vi "Wireless Logging Example.vi"() -> ()   [LabVIEW 2024]
uses:
  Log Levels.ctl
  Failure Information.ctl
  Log Record.ctl
  Logger/Internal Log Levels.ctl
  ff44e4a9-c346-414c-ae2a-efcf3ff82913.vi
  0679c0b6-e665-4267-8d21-5c2f63ff0cfc.vi
  b68c178a-45ff-4a43-8ee1-f997d7190e6c.vi
  26cdefab-9c11-46d6-bea8-26d872e8373c.vi
  cd3cbcb6-eea4-4d7a-90d3-75033959401d.vi
  3aace37d-2631-4088-b4d1-fd5fc03c86bc.vi
  0679c0b6-e665-4267-8d21-5c2f63ff0cfc.vi/a153a250-4fb8-4a99-bb5b-6ccb57f1f631.vi
  b68c178a-45ff-4a43-8ee1-f997d7190e6c.vi/a02c6254-97f5-44e3-a3a9-7fdb6dfbd055.vi
  26cdefab-9c11-46d6-bea8-26d872e8373c.vi/bae24b8d-f663-491e-8374-2218e527d0d0.vi
  cd3cbcb6-eea4-4d7a-90d3-75033959401d.vi/bf655d3c-1ce4-400f-a78f-0f3f0191886e.vi
  Mark Error.vi
  3aace37d-2631-4088-b4d1-fd5fc03c86bc.vi/ba94d47b-0e30-4c32-b8ff-86d609cd95a5.vi
  0679c0b6-e665-4267-8d21-5c2f63ff0cfc.vi/a153a250-4fb8-4a99-bb5b-6ccb57f1f631.vi/28727e37-b0d9-407c-a479-ab0b7779cd69.vi
  b68c178a-45ff-4a43-8ee1-f997d7190e6c.vi/a02c6254-97f5-44e3-a3a9-7fdb6dfbd055.vi/7453dcce-b283-4a0d-ab92-51c518b086c4.vi
  26cdefab-9c11-46d6-bea8-26d872e8373c.vi/bae24b8d-f663-491e-8374-2218e527d0d0.vi/083db1d9-8cf1-45e4-a540-e8e178cc7cc8.vi
  Handlers/String Handler/String Handler.lvclass
  Formatters/JSON/JSON.lvclass
  <vilib>/Utility/error.llb/Error Cluster From Error Code.vi
  Registry/Enable All.vi
  Registry/Disable All.vi
  Registry/Log.vi
  <vilib>/ErrorRing/Error Ring.xnode
  C:/Users/Colin/Documents/software_projects/glog/Logging/Handlers/Formatting Handler/Formatting Handler.lvclass
  C:/Users/Colin/Documents/software_projects/glog/Logging/Handlers/String Handler/String Handler.lvclass
  Logging.lvlib
  C:/Users/Colin/Documents/software_projects/glog/Logging/Formatters/Formatter/Formatter.lvclass
  C:/Users/Colin/Documents/software_projects/glog/Logging/Formatters/JSON/JSON.lvclass
panel:
  in  "Failure Type":bool
  out "failures info":T1[](array[typedef]) {"Log Record"."timestamp" format="%<%x %.3X>T"}
  in  "error/warning iteration":i32=20
  in  "log messages 2":string
  in  "loop iteration delay [ms]":u32=10
  in  "minimum log level":T4=enum."Info"
  out "error out":errorcluster
  in  "log messages":string
  in  "total iterations":i32=30
  in  "restart logging at":i32=20
  in  "stop logging at":i32=10
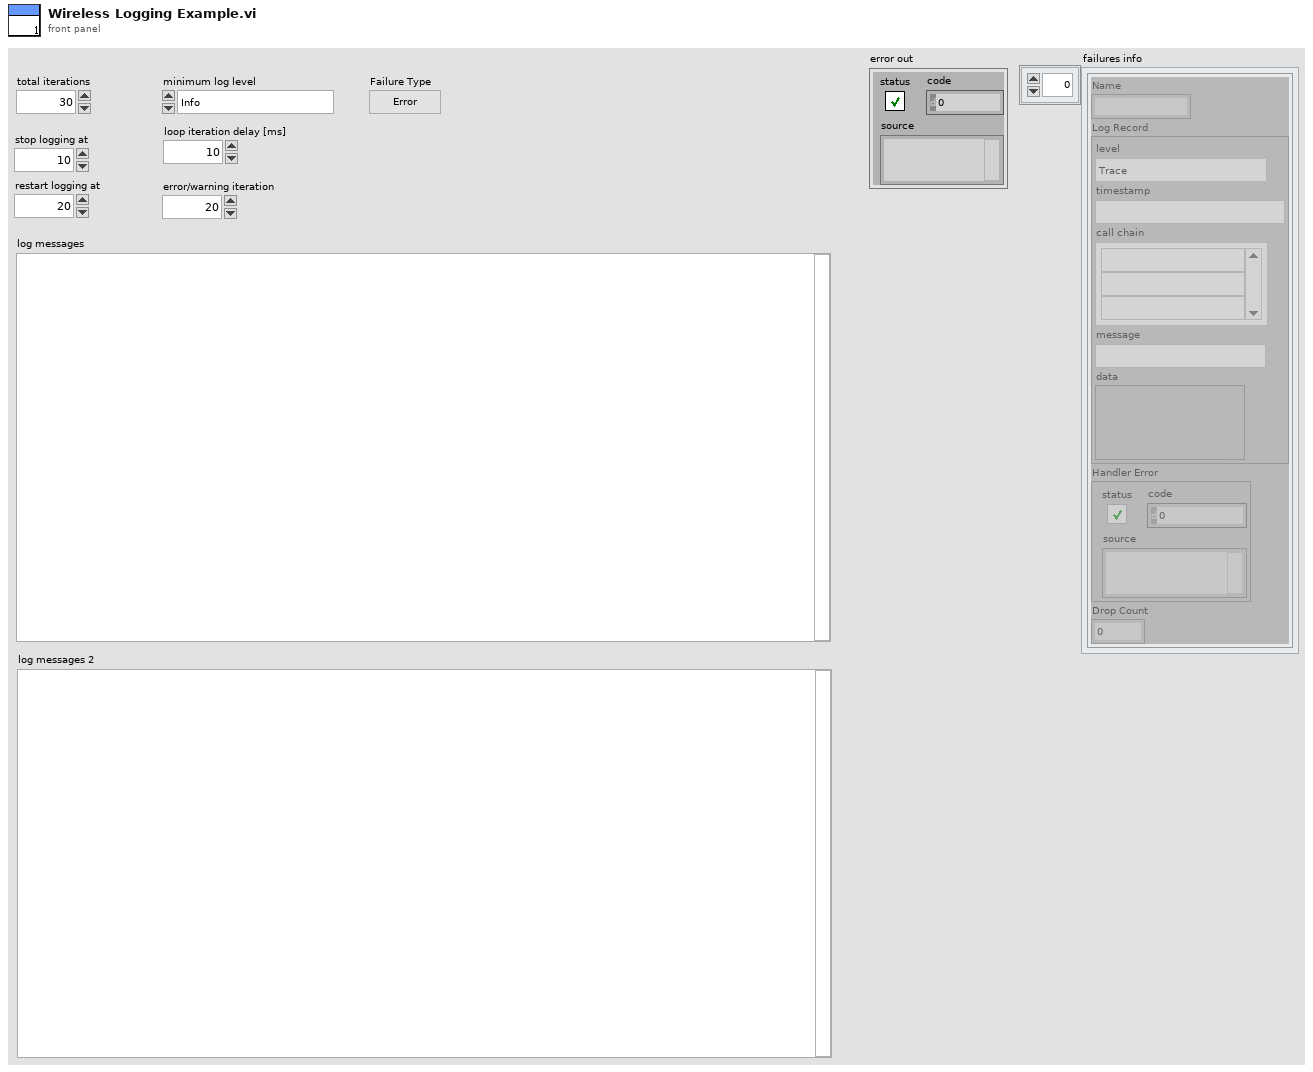
[diagram p1: front panel]
types:
  T1 = typedef "Logging.lvlib/Failure Information.ctl" = cluster{"Name":string, "Log Record":T2, "Handler Error":errorcluster, "Drop Count":u32}
  T2 = typedef "Logging.lvlib/Log Record.ctl" = cluster{"level":T3, "timestamp":timestamp, "call chain":string[], "message":string, "data":variant}
  T3 = typedef "Logging.lvlib/Internal Log Levels.ctl" = enum16{"Trace", "Debug", "Info", "Warning", "Error", "Critical", "Internal"}
  T4 = typedef "Logging.lvlib/Log Levels.ctl" = enum16{"Trace", "Debug", "Info", "Warning", "Error", "Critical"}
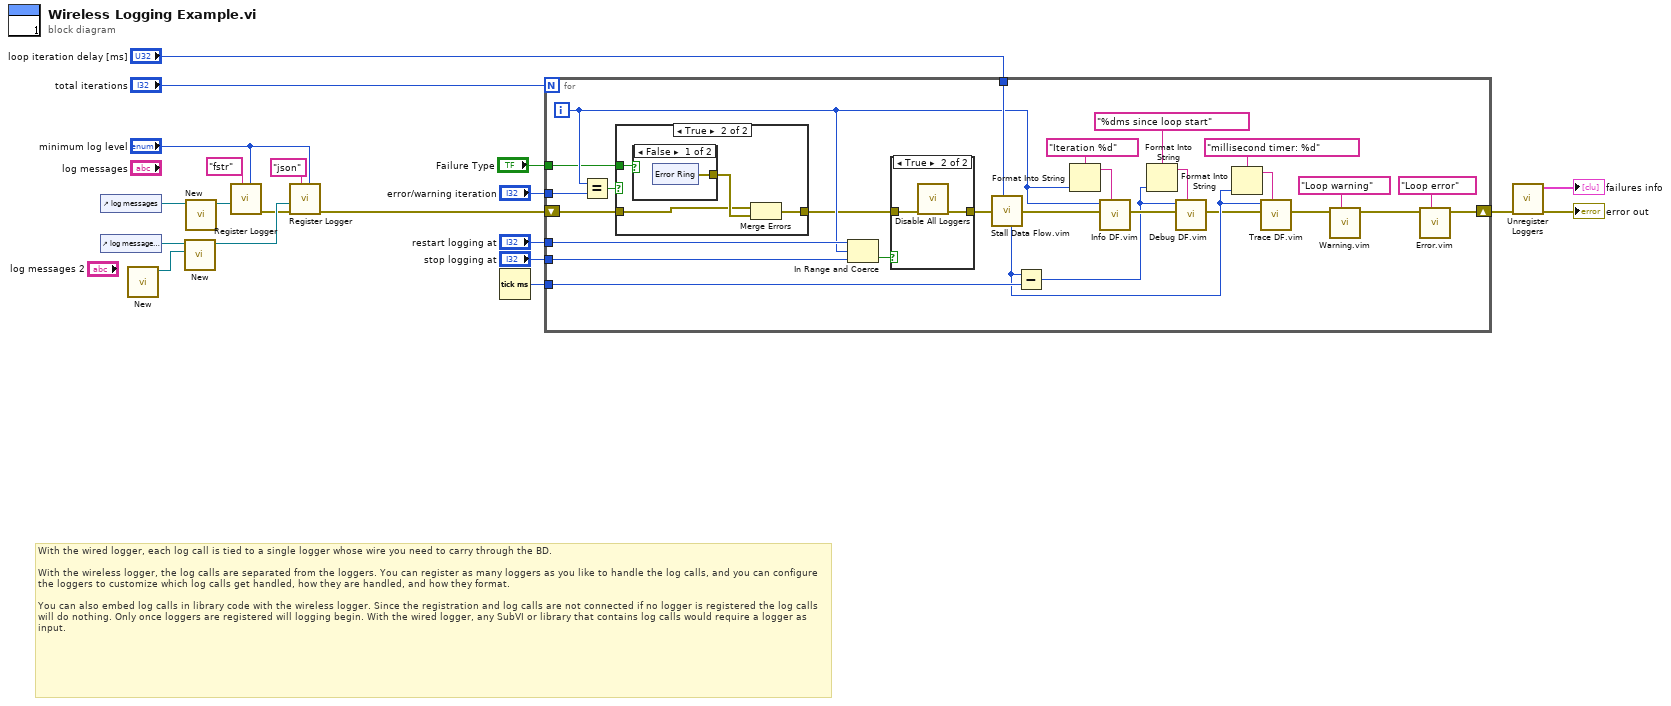
[diagram p0: block diagram]
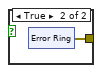
[diagram p3: hidden frame]
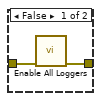
[diagram p4: hidden frame]
diagram:
  # "With the wired logger, each log call is tied to a single logger whose wire you need to carry through the BD.\n\nWith the wireless logger, the log calls are separated from the loggers. You can register as many loggers as you like to handle the log calls, and you can configure the loggers to customize which log calls get handled, how they are handled, and how they format.\n\nYou can also embed log calls in library code with the wireless logger. Since the registration and log calls are not connected if no logger is registered the log calls will do nothing. Only once loggers are registered will logging begin. With the wired logger, any SubVI or library that contains log calls would require a logger as input."
  n1 = control-ref of="log messages"() -> (w15:refnum<vi>)
  n2 = control-ref of="log messages 2"() -> (w12:refnum<vi>)
  n3 = call "New.vi"() -> ("JSON formatter"=w10:refnum<class "JSON.lvclass">)  [unwired: 11 in]
  n4 = call "New.vi"("formatter (format string)"=w10, "string control"=w12) -> ("new string handler"=w11:refnum<class "String Handler.lvclass">)  [unwired: 9 in]
  n5 = call "New.vi"("string control"=w15) -> ("new string handler"=w16:refnum<class "String Handler.lvclass">)  [unwired: 10 in]
  n6 = call "Register Logger.vi"("minimum log level (Info)"="minimum log level", "name (\"Default\")"="fstr" ("name (\"Default\")"), "log handler (file handler)"=w16) -> ("error out"=w4:errorcluster)  [unwired: 8 in]
  n7 = call "Register Logger.vi"("minimum log level (Info)"="minimum log level", "name (\"Default\")"="json" ("name (\"Default\")"), "error in (no error)"=w4, "log handler (file handler)"=w11) -> ("error out"=w3:errorcluster)  [unwired: 7 in]
  n8 = Tick Count (ms)() -> (millisecond timer value=w20:u32)
  n9 = for {
    N: "total iterations" -> [_]
    tunnel: w20 -> [w48]
    tunnel: "stop logging at" -> [w46]
    tunnel: "restart logging at" -> [w45]
    shift-right: [w31] -> w1
    shift-left: w3 -> [w26]
    tunnel: "loop iteration delay [ms]" -> [w43]
    tunnel: "error/warning iteration" -> [w28]
    tunnel: "Failure Type" -> [w21]
    i -> [w29]
    n10 = Equal?(x=w29, y=w28) -> (x = y?=w27:bool)
    n11 = case shown="True" w27 {
      tunnel: w26 -> [w49 w51]
      tunnel: [w49 w52] -> w25
      tunnel: w21 -> [_ w50]
      frame False {
      }
      frame True {
        n12 = case shown="False" w50 {
          tunnel: [w54 w60] -> w53
          frame False {
            n13 = xnode "Error Ring"() -> ("error out"=w54:errorcluster)
          }
          frame True {
            n14 = xnode "Error Ring"() -> ("error out"=w60:errorcluster)
          }
        }
        n15 = Merge Errors(w51, w53) -> (w52:errorcluster)
      }
    }
    n16 = In Range and Coerce(upper limit=w45, x=w29, lower limit=w46) -> (In Range?=w47:bool)  [unwired: 1 out]
    n17 = case shown="True" w47 {
      tunnel: w25 -> [w67 w69]
      tunnel: [w66 w68] -> w42
      frame False {
        n18 = call "Enable All Loggers.vi"("error in"=w67) -> ("error out"=w66:errorcluster)  [unwired: 10 in]
      }
      frame True {
        n19 = call "Disable All Loggers.vi"("error in"=w69) -> ("error out"=w68:errorcluster)  [unwired: 10 in]
      }
    }
    n20 = call "Stall Data Flow.vim"("value in"=w42, "milliseconds to wait"=w43) -> ("millisecond timer value"=w33:u32, "value out"=w41:errorcluster)
    n21 = Subtract(x=w33, y=w48) -> (x-y=w37:u32)
    n22 = Format Into String(format string="Iteration %d" ("message"), w29) -> (resulting string=w40:string)  [unwired: 2 in, 1 out]
    n23 = call "Info DF.vim"("message"=w40, "dataflow in"=w41, "data (null)"=w29) -> ("dataflow out"=w38:errorcluster)  [unwired: 8 in]
    n24 = Format Into String(format string="%dms since loop start" ("message"), w37) -> (resulting string=w39:string)  [unwired: 2 in, 1 out]
    n25 = call "Debug DF.vim"("message"=w39, "dataflow in"=w38, "data (null)"=w37) -> ("dataflow out"=w32:errorcluster)  [unwired: 8 in]
    n26 = Format Into String(format string="millisecond timer: %d" ("message"), w33) -> (resulting string=w34:string)  [unwired: 2 in, 1 out]
    n27 = call "Trace DF.vim"("message"=w34, "dataflow in"=w32, "data (null)"=w33) -> ("dataflow out"=w24:errorcluster)  [unwired: 8 in]
    n28 = call "Warning.vim"("data in (null)"=w24, "message"="Loop warning") -> ("data out"=w23:errorcluster)  [unwired: 9 in]
    n29 = call "Error.vim"("data in (null)"=w23, "message"="Loop error") -> ("data out"=w31:errorcluster)  [unwired: 9 in]
  }
  n30 = call "Unregister Loggers.vi"("error in (no error)"=w1) -> ("error out"=→"error out":errorcluster, "failures info"=→"failures info":T1[])  [unwired: 9 in]
